vi "AppendFrontPanelImageToReportOldString_Mutation.vi"(0 "Diagram":refnum<vi>, 5 "ObjRef":refnum<vi>, 6 "Kind":string="SubVI", 7 "Information":string="<Not A Path>") -> (3 "Replace?":bool)   [LabVIEW 2020]
uses:
  <vilib>/Utility/miscctls.llb/LVPositionTypeDef.ctl
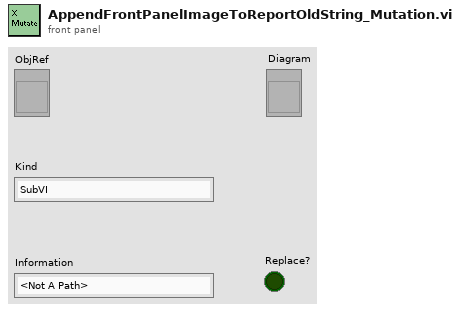
[diagram p1: front panel]
types:
  T1 = typedef "LVPositionTypeDef.ctl" = cluster{"Left":i32, "Top":i32}
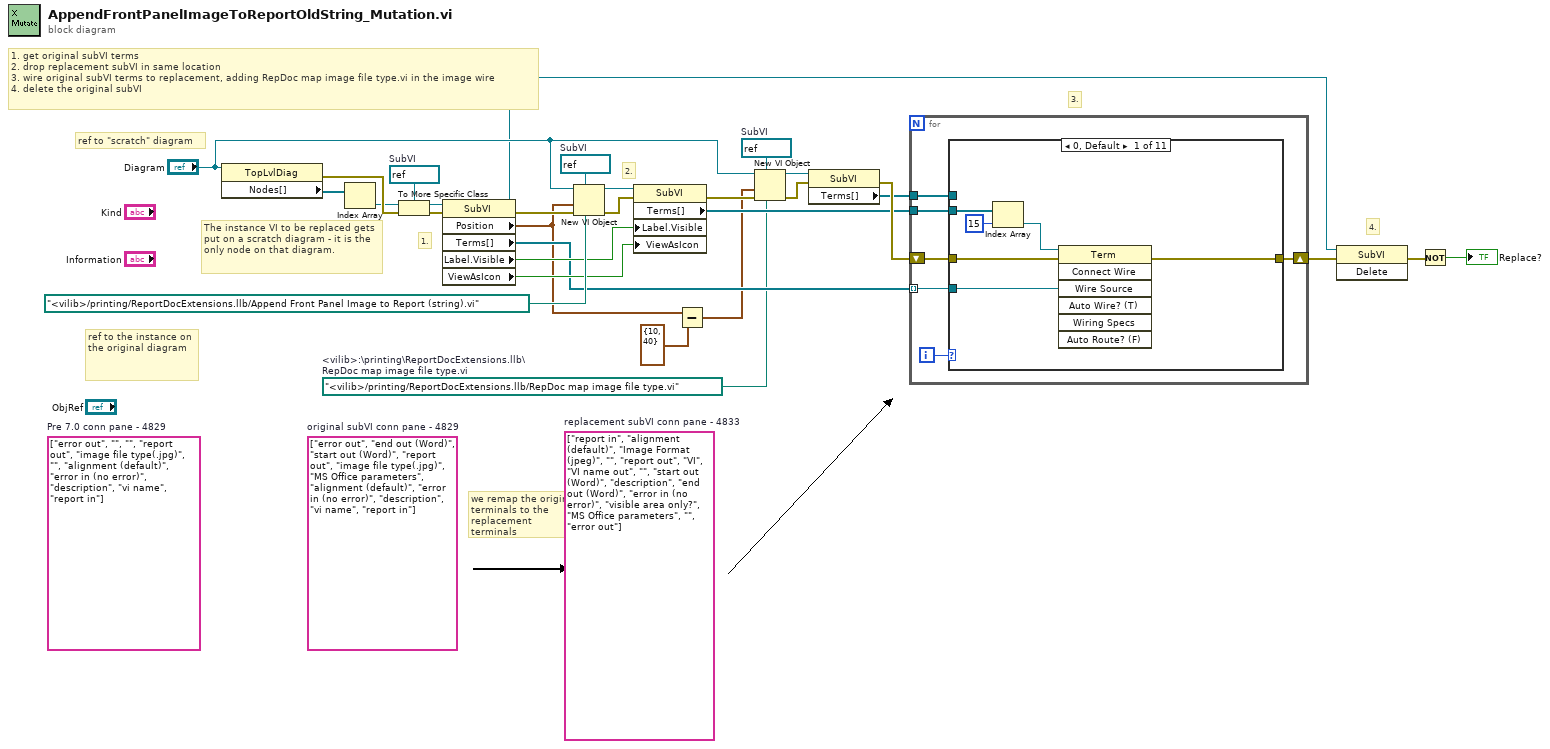
[diagram p0: block diagram]
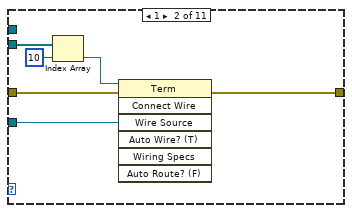
[diagram p2: hidden frame]
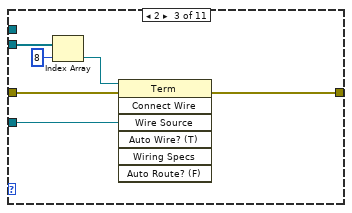
[diagram p3: hidden frame]
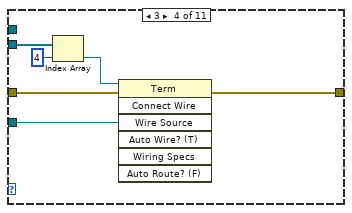
[diagram p4: hidden frame]
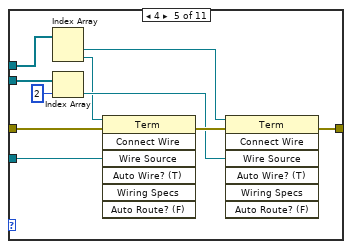
[diagram p5: hidden frame]
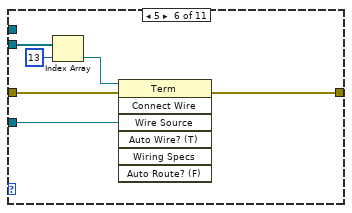
[diagram p6: hidden frame]
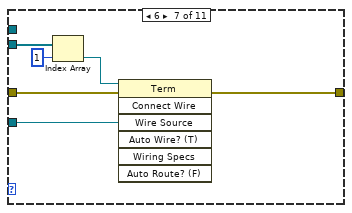
[diagram p7: hidden frame]
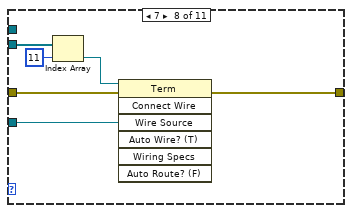
[diagram p8: hidden frame]
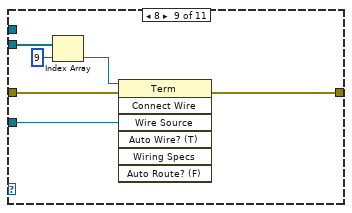
[diagram p9: hidden frame]
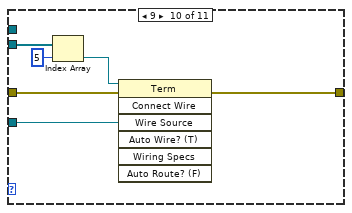
[diagram p10: hidden frame]
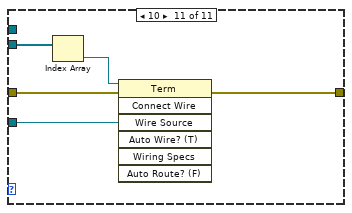
[diagram p11: hidden frame]
diagram:
  (unwired) string[] ["error out", "", "", "report out", "image file type(.jpg)", "", "alignment (default)", "error in (no error)", "description", "vi name", "report in"]  # Pre 7.0 conn pane - 4829
  w10 = refnum<vi> refnum  # SubVI
  w9 = path "<vilib>/printing/ReportDocExtensions.llb/RepDoc map image file type.vi"  # <vilib>:\printing\ReportDocExtensions.llb\RepDoc map image file type.vi
  (unwired) string[] ["report in", "alignment (default)", "Image Format (jpeg)", "", "report out", "VI", "VI name out", "", "start out (Word)", "description", "end out (Word)", "error in (no error)", "visible area only?", "MS Office parameters", "", "error out"]  # replacement subVI conn pane - 4833
  (unwired) string[] ["error out", "end out (Word)", "start out (Word)", "report out", "image file type(.jpg)", "MS Office parameters", "alignment (default)", "error in (no error)", "description", "vi name", "report in"]  # original subVI conn pane - 4829
  w19 = refnum<vi> refnum  # SubVI
  w21 = refnum<vi> refnum  # SubVI
  # "4."
  # "3."
  # "2."
  # "1."
  # "we remap the original terminals to the replacement terminals"
  # "The instance VI to be replaced gets put on a scratch diagram - it is the only node on that diagram."
  # "1. get original subVI terms\n2. drop replacement subVI in same location\n3. wire original subVI terms to replacement, adding RepDoc map image file type.vi in the image wire\n4. delete the original subVI"
  # "ref to the instance on the original diagram"
  # "ref to \"scratch\" diagram"
  n1 = property class="TopLvlDiag"(reference="Diagram") -> (error out=w26:errorcluster, "Nodes[]"=w18:refnum<vi>[])  [unwired: 1 in, 1 out]
  n2 = Index Array(array=w18) -> (element=w17:refnum<vi>)  [unwired: 1 in]
  n3 = To More Specific Class(target class=w21, reference=w17, error in=w26) -> (specific class reference=w20:refnum<vi>, error out=w30:errorcluster)
  n4 = property class="SubVI"(reference=w20, error in=w30) -> (reference out=w3:refnum<vi>, error out=w24:errorcluster, "Position"=w7:T1, "Terms[]"=w12:refnum<vi>[], "Label.Visible"=w14:bool, "ViewAsIcon"=w13:bool)
  n5 = New VI Object(vi object class=w19, owner refnum="Diagram", position/next to=w7, 6:path "<vilib>/printing/ReportDocExtensions.llb/Append Front Panel Image to Report (string).vi", 8:w24) -> (object refnum=w15:refnum<vi>, 0:w23:errorcluster)  [unwired: 3 in]
  n6 = property class="SubVI"(reference=w15, error in=w23, "Label.Visible"=w14, "ViewAsIcon"=w13) -> (error out=w29:errorcluster, "Terms[]"=w11:refnum<vi>[])  [unwired: 1 out]
  n7 = Subtract(x=w7, y=T1 {"Left"=10, "Top"=40}) -> (x-y=w6:T1)
  n8 = New VI Object(vi object class=w10, owner refnum="Diagram", position/next to=w6, 6:w9, 8:w29) -> (object refnum=w4:refnum<vi>, 0:w25:errorcluster)  [unwired: 3 in]
  n9 = property class="SubVI"(reference=w4, error in=w25) -> (error out=w27:errorcluster, "Terms[]"=w1:refnum<vi>[])  [unwired: 1 out]
  n10 = for {
    tunnel: w12 -> [w33] mode=indexing
    tunnel: w11 -> [w32]
    shift-right: [w35] -> w28
    shift-left: w27 -> [w36]
    tunnel: w1 -> [w31]
    i -> [w34]
    n11 = case shown="0, Default" w34 {
      tunnel: w33 -> [w40 w46 w52 w58 w67 w74 w80 w86 w92 w98 w103]
      tunnel: w32 -> [w39 w45 w51 w57 w66 w73 w79 w85 w91 w97 w102]
      tunnel: w36 -> [w42 w48 w54 w60 w70 w76 w82 w88 w94 w100 w105]
      tunnel: [w41 w47 w53 w59 w68 w75 w81 w87 w93 w99 w104] -> w35
      tunnel: w31 -> [_ _ _ _ w64 _ _ _ _ _ _]
      frame 0, Default {
        n12 = Index Array(array=w39, index=15) -> (element=w37:refnum<vi>)
        n13 = invoke class="Term" method="Connect Wire"(reference=w37, error in=w42, "Wire Source"=w40) -> (error out=w41:errorcluster)  [unwired: 4 in, 6 out]
      }
      frame 1 {
        n14 = Index Array(array=w45, index=10) -> (element=w43:refnum<vi>)
        n15 = invoke class="Term" method="Connect Wire"(reference=w43, error in=w48, "Wire Source"=w46) -> (error out=w47:errorcluster)  [unwired: 4 in, 6 out]
      }
      frame 2 {
        n16 = Index Array(array=w51, index=8) -> (element=w49:refnum<vi>)
        n17 = invoke class="Term" method="Connect Wire"(reference=w49, error in=w54, "Wire Source"=w52) -> (error out=w53:errorcluster)  [unwired: 4 in, 6 out]
      }
      frame 3 {
        n18 = Index Array(array=w57, index=4) -> (element=w55:refnum<vi>)
        n19 = invoke class="Term" method="Connect Wire"(reference=w55, error in=w60, "Wire Source"=w58) -> (error out=w59:errorcluster)  [unwired: 4 in, 6 out]
      }
      frame 4 {
        n20 = Index Array(array=w64) -> (element #1=w63:refnum<vi>, element #2=w61:refnum<vi>)  [unwired: 2 in]
        n21 = Index Array(array=w66, index=2) -> (element=w62:refnum<vi>)
        n22 = invoke class="Term" method="Connect Wire"(reference=w61, error in=w70, "Wire Source"=w67) -> (error out=w69:errorcluster)  [unwired: 4 in, 6 out]
        n23 = invoke class="Term" method="Connect Wire"(reference=w63, error in=w69, "Wire Source"=w62) -> (error out=w68:errorcluster)  [unwired: 4 in, 6 out]
      }
      frame 5 {
        n24 = Index Array(array=w73, index=13) -> (element=w71:refnum<vi>)
        n25 = invoke class="Term" method="Connect Wire"(reference=w71, error in=w76, "Wire Source"=w74) -> (error out=w75:errorcluster)  [unwired: 4 in, 6 out]
      }
      frame 6 {
        n26 = Index Array(array=w79, index=1) -> (element=w77:refnum<vi>)
        n27 = invoke class="Term" method="Connect Wire"(reference=w77, error in=w82, "Wire Source"=w80) -> (error out=w81:errorcluster)  [unwired: 4 in, 6 out]
      }
      frame 7 {
        n28 = Index Array(array=w85, index=11) -> (element=w83:refnum<vi>)
        n29 = invoke class="Term" method="Connect Wire"(reference=w83, error in=w88, "Wire Source"=w86) -> (error out=w87:errorcluster)  [unwired: 4 in, 6 out]
      }
      frame 8 {
        n30 = Index Array(array=w91, index=9) -> (element=w89:refnum<vi>)
        n31 = invoke class="Term" method="Connect Wire"(reference=w89, error in=w94, "Wire Source"=w92) -> (error out=w93:errorcluster)  [unwired: 4 in, 6 out]
      }
      frame 9 {
        n32 = Index Array(array=w97, index=5) -> (element=w95:refnum<vi>)
        n33 = invoke class="Term" method="Connect Wire"(reference=w95, error in=w100, "Wire Source"=w98) -> (error out=w99:errorcluster)  [unwired: 4 in, 6 out]
      }
      frame 10 {
        n34 = Index Array(array=w102) -> (element=w101:refnum<vi>)  [unwired: 1 in]
        n35 = invoke class="Term" method="Connect Wire"(reference=w101, error in=w105, "Wire Source"=w103) -> (error out=w104:errorcluster)  [unwired: 4 in, 6 out]
      }
    }
  }
  n36 = invoke class="SubVI" method="Delete"(reference=w3, error in=w28) -> (error out=w22:errorcluster)  [unwired: 1 in, 2 out]
  n37 = Not(x=w22) -> (.not. x?=→"Replace?":bool)
